vi "oa_Shift and Low Pass Filter (1 Channel, Obsolete).vi"(0 "input signal":dbl[](array[numeric]), 1 "reset? (F)":bool, 5 "t0":dbl, 7 "center":dbl, 9 "decimation factor":u32, 11 "error in (no error)":errorcluster, 12 "new dt":dbl) -> (4 "enveloped signal":dbl[](array[numeric]), 6 "t0 out":dbl, 15 "error out":errorcluster)   [LabVIEW 2017]
uses:
  <vilib>/addons/Sound and Vibration/Order Analysis/Adv Resampling/OAT Single Stage Decimation with IC.vi
  <vilib>/addons/Sound and Vibration/Order Analysis/Resample Order Tracking/SubVIs/OAT CIC Decimation.vi
  <vilib>/addons/Sound and Vibration/Order Analysis/Resample Order Tracking/SubVIs/oa_Interpolate Zeros Between Samples.vi
  <vilib>/addons/Sound and Vibration/Order Analysis/Resample Order Tracking/SoundVib_Resampling.lvlib
  <vilib>/Analysis/NI_AALPro.lvlib
  <vilib>/addons/Sound and Vibration/Order Analysis/Fault Analysis/SoundVib_FaultAnalysis.lvlib
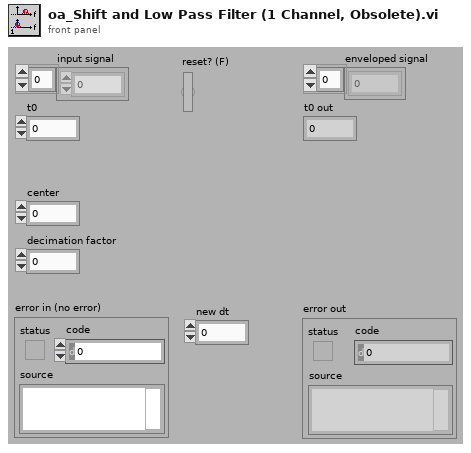
[diagram p1: front panel]
types:
  T1 = typedef "OAT Decimation Filter.ctl" = cluster{"coefficients":dbl[], "factor":i32}
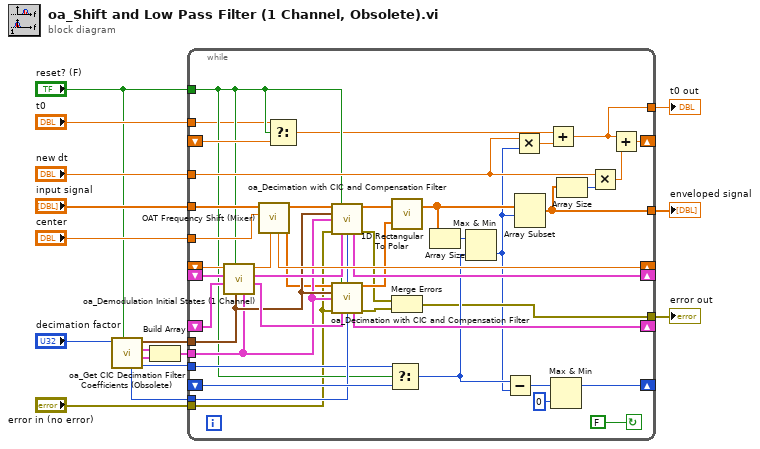
[diagram p0: block diagram]
diagram:
  n1 = call <vilib>:"oa_Get CIC Decimation Filter Coefficients (Obsolete).vi"("reset? (True)"="reset? (F)", "decimation/interpolation factor"="decimation factor") -> ("delay"=w11:i32, "lp filter settings"=w14:T1, "compensation filter settings"=w15:T1, "CIC Settings"=w16:cluster{"Numeric":i32, i32, i32}, "interpolation factor"=w12:i32)  [unwired: 5 in]
  n2 = Build Array(w15, w14) -> (w13:T1[])
  n3 = while {
    shift-left: _ -> [w55]
    shift-right: [w56] -> _
    shift-left: _ -> [w47]
    shift-right: [w49] -> _
    shift-left: _ -> [w46]
    shift-right: [w48] -> _
    tunnel: "center" -> [w58]
    tunnel: "input signal" -> [w59]
    tunnel: [w36] -> w10
    tunnel: [w31] -> w8
    shift-right: [w50] -> _
    shift-left: _ -> [w53]
    tunnel: w16 -> [w43]
    tunnel: w13 -> [w41]
    tunnel: w12 -> [w42]
    tunnel: w11 -> [w40]
    shift-right: [w33] -> _
    shift-left: _ -> [w37]
    tunnel: "t0" -> [w20]
    tunnel: "new dt" -> [w32]
    tunnel: "reset? (F)" -> [w22]
    tunnel: [w18] -> w3
    tunnel: "error in (no error)" -> [w21]
    stop <- FALSE continue-if-true
    n4 = call <vilib>:"oa_Demodulation Initial States (1 Channel).vi"("filters"=w41, "CIC filter settings"=w43, "reset? (F)"=w22, "imaginary state in"=w46, "real state in"=w47, "phase in"=w55) -> ("imaginary state out"=w44:cluster{cluster{dbl[]}, cluster{dbl[]}[]}, "real state out"=w45:cluster{cluster{dbl[]}, cluster{dbl[]}[]}, "phase out"=w54:dbl)  [unwired: 3 in]
    n5 = call <vilib>:"OAT Frequency Shift (Mixer).vi"("initial phase"=w54, "fc"=w58, "X"=w59) -> ("imaginary"=w29:dbl[], "real"=w26:dbl[], "final phase"=w56:dbl)  [unwired: 6 in]
    n6 = Select(t=w20, s=w22, f=w37) -> (s? t:f=w19:dbl)
    n7 = call <vilib>:"oa_Decimation with CIC and Compensation Filter.vi"("x[n]"=w26, "reset? (True)"=w22, "CIC decimation setting"=w43, "decimation filters"=w41, "error in (no error)"=w21, "statein"=w45, "interpolation factor"=w42) -> ("x[n] out"=w24:dbl[], "state out"=w49:cluster{cluster{dbl[]}, cluster{dbl[]}[]}, "error out"=w25:errorcluster)  [unwired: 6 in]
    n8 = call <vilib>:"oa_Decimation with CIC and Compensation Filter.vi"("x[n]"=w29, "reset? (True)"=w22, "CIC decimation setting"=w43, "decimation filters"=w41, "error in (no error)"=w21, "statein"=w44, "interpolation factor"=w42) -> ("x[n] out"=w30:dbl[], "state out"=w48:cluster{cluster{dbl[]}, cluster{dbl[]}[]}, "error out"=w28:errorcluster)  [unwired: 6 in]
    n9 = Select(t=w40, s=w22, f=w53) -> (s? t:f=w39:i32)
    n10 = call <vilib>:"1D Rectangular To Polar.vi"("X"=w24, "Y"=w30) -> ("Magnitude"=w23:dbl[])  [unwired: 2 out]
    n11 = Merge Errors(w25, w28) -> (w31:errorcluster)
    n12 = Array Size(array=w23) -> (size(s)=w27:i32)
    n13 = Max & Min(x=w27, y=w39) -> (min(x,y)=w17:i32)  [unwired: 1 out]
    n14 = Subtract(x=w39, y=w17) -> (x-y=w52:i32)
    n15 = Multiply(x=w32, y=w17) -> (x*y=w38:dbl)
    n16 = Array Subset(array=w23, index=w17) -> (w36:dbl[])  [unwired: 1 in]
    n17 = Add(x=w19, y=w38) -> (x+y=w18:dbl)
    n18 = Max & Min(x=w52, y=0) -> (max(x,y)=w50:i32)  [unwired: 1 out]
    n19 = Array Size(array=w36) -> (size(s)=w35:i32)
    n20 = Multiply(x=w32, y=w35) -> (x*y=w34:dbl)
    n21 = Add(x=w18, y=w34) -> (x+y=w33:dbl)
  }
  "error out" <- w8
  "enveloped signal" <- w10
  "t0 out" <- w3
